vi "Read Dispatcher Error.vi"(8 "error in (no error)":errorcluster, 9 "timeout in ms (0)":i32 format="%d ms", 11 "Dispatcher Interface in":refnum<class "Dispatcher Interface.lvclass">) -> (0 "error out":errorcluster, 2 "error":errorcluster, 3 "Dispatcher Interface out":refnum<class "Dispatcher Interface.lvclass">)   [LabVIEW 2019, in "DSF Core.lvlib" / "Dispatcher Interface.lvclass"]
uses:
  Dispatcher Interface.lvclass
  C:/Dev/GitHub/niveristand-data-sharing-framework-custom-device/Core/Classes/Interface/Interface.lvclass
  Error Timeout.vi
  Interface.lvclass
  DSF Core.lvlib
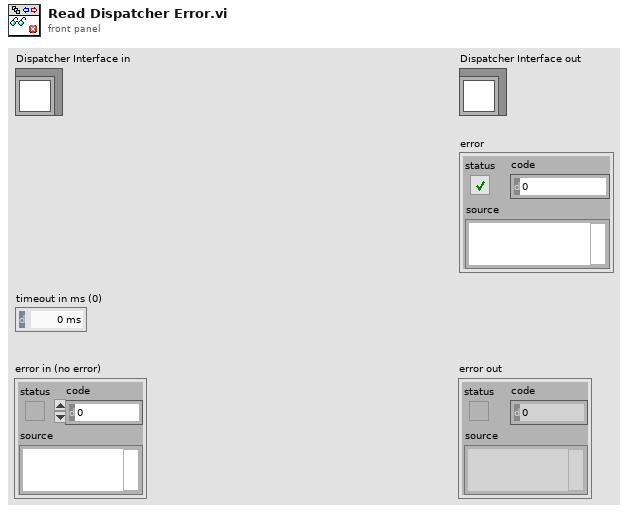
[diagram p1: front panel]
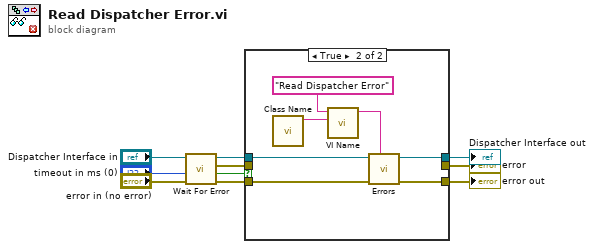
[diagram p0: block diagram]
diagram:
  n1 = call "Wait For Error.vi"("error in (no error)"="error in (no error)", "timeout in ms (0)"="timeout in ms (0)", "Interface in"="Dispatcher Interface in") -> ("error out"=w6:errorcluster, "timed out?"=w7:bool, "error"=w5:errorcluster, "Interface out"=w4:refnum<class "Dispatcher Interface.lvclass">)  [unwired: 4 in, 1 out]
  n2 = case shown="True" w7 {
    tunnel: w6 -> [w12 w19]
    tunnel: w5 -> [w11 _]
    tunnel: w4 -> [w13 w20]
    tunnel: [w13 w18] -> w3
    tunnel: [w12 w17] -> w2
    tunnel: [w11 _] -> w1
    frame False {
    }
    frame True {
      n3 = call "Class Name.vi"() -> ("class name"=w16:string)  [unwired: 11 in]
      n4 = call "VI Name.vi"("class name (\"\")"=w16, "vi name"="Read Dispatcher Error" ("error source vi name")) -> ("full VI name"=w14:string)  [unwired: 9 in]
      n5 = call-poly "Errors.vi"("error source vi name"=w14, "error in (no error)"=w19, "Interface in"=w20) -> ("error out"=w17:errorcluster, "Interface out"=w18:refnum<class "Dispatcher Interface.lvclass">)  [unwired: 7 in]
    }
  }
  "error out" <- w2
  "Dispatcher Interface out" <- w3
  "error" <- w1
